vi "Unloading Sequence.vi"(8 "Abort":bool, 11 "Unload Button":bool) -> (0 "Not Start":bool)   [LabVIEW 2014]
uses:
  Unload State.ctl
  2015/2015 Master Code RECYCLE RUSH/Robot Global Data.vi
  Desired Arm Position.vi
panel:
  in  "Parameter":T1
  out "Turn 180":bool
  out "Close Arms":bool
  out "Open Arms":bool
  out "Lower Back Arms":bool
  out "Move Back":bool
  out "Raise Arms":bool
  out "Unload Front Arms":bool
  out "Start":bool
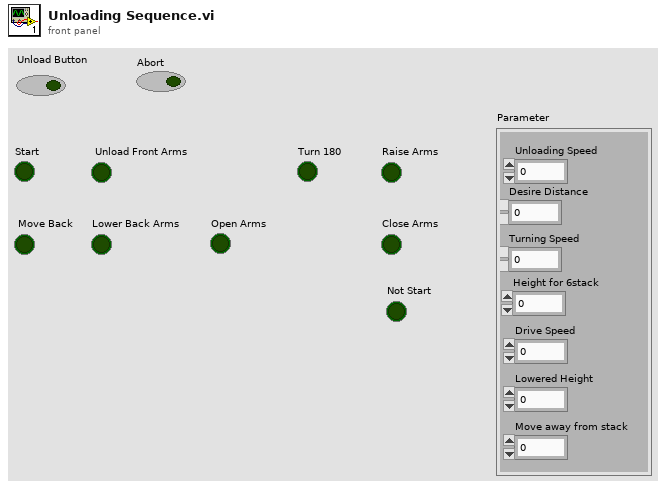
[diagram p1: front panel]
types:
  T1 = cluster{"Desire Distance  ":dbl, "Turning Speed":dbl, "Height for 6stack":dbl, "Drive Speed":dbl, "Lowered Height":dbl, "Move away from stack":dbl, "Unloading Speed":dbl}
  T2 = typedef "Unload State.ctl" = enum16{"Start", "Unload", "Back up", "Turn 180", "Raise Arms", "Move Back to S.P.", "Lower Back Arms", "Open Arms", "Back Up Before Drive", "Close Arms"}
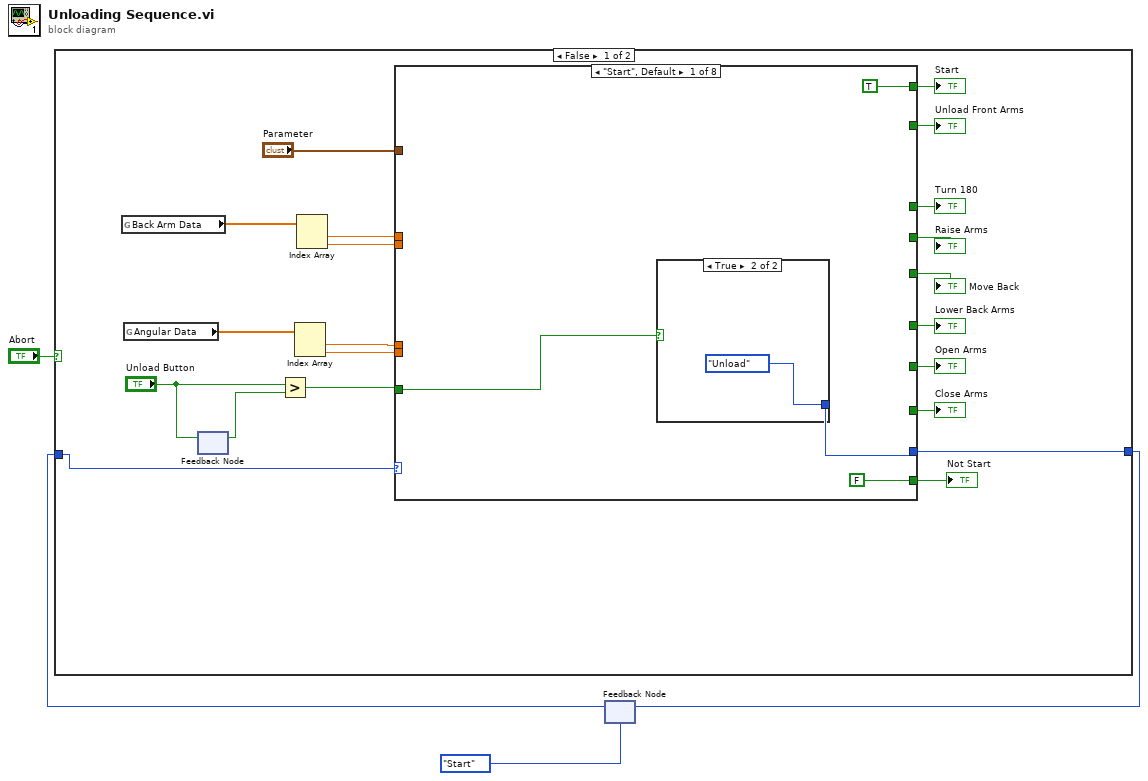
[diagram p0: block diagram]
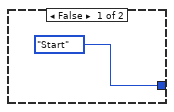
[diagram p2: hidden frame]
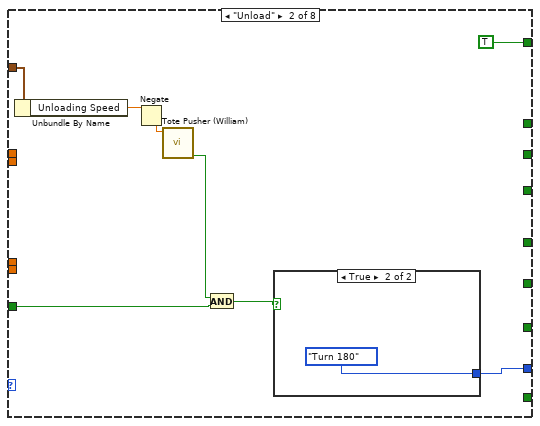
[diagram p3: hidden frame]
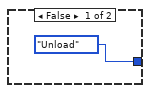
[diagram p4: hidden frame]
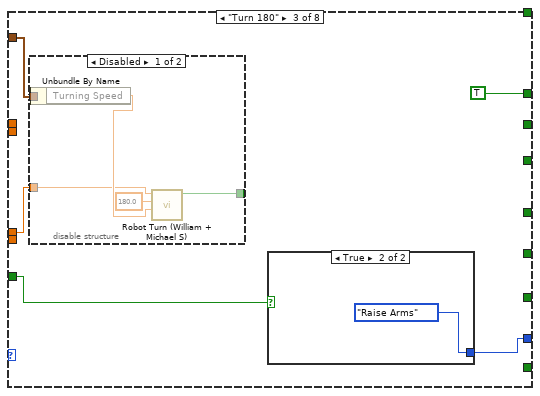
[diagram p5: hidden frame]
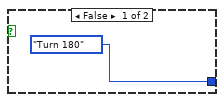
[diagram p7: hidden frame]
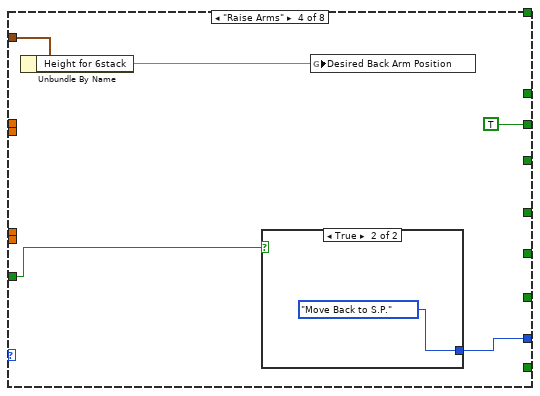
[diagram p8: hidden frame]
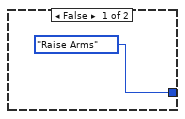
[diagram p9: hidden frame]
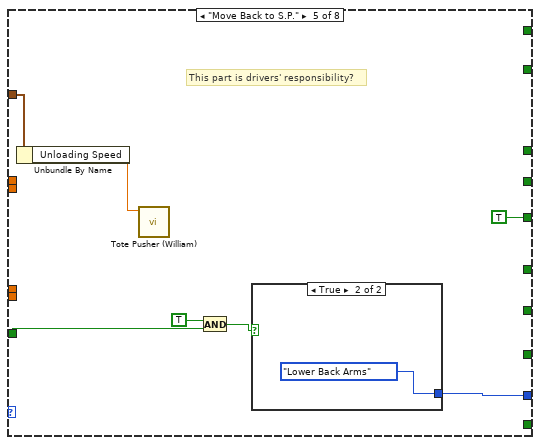
[diagram p10: hidden frame]
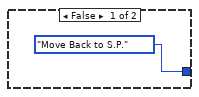
[diagram p11: hidden frame]
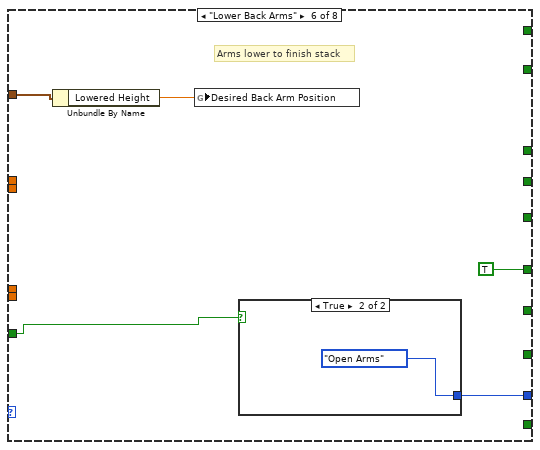
[diagram p12: hidden frame]
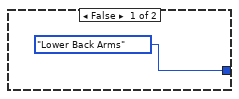
[diagram p13: hidden frame]
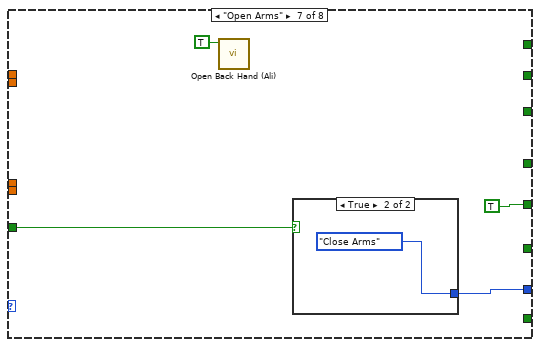
[diagram p14: hidden frame]
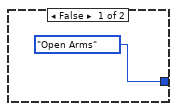
[diagram p15: hidden frame]
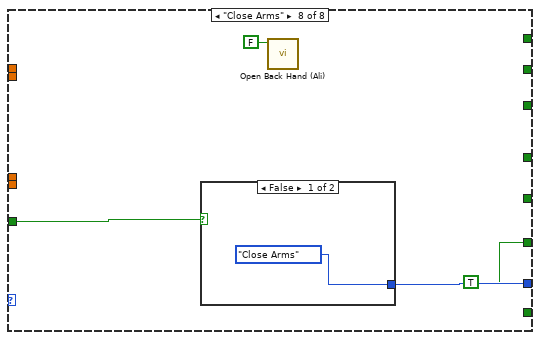
[diagram p16: hidden frame]
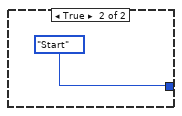
[diagram p17: hidden frame]
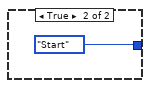
[diagram p18: hidden frame]
diagram:
  n1 = feedback #1(Unload_State."Start") -> (w2:T2)
  n2 = case shown="False" "Abort" {
    tunnel: [w7 Unload_State."Start"] -> w3
    tunnel: w2 -> [w6 _]
    frame False {
      n3 = global read "Robot Global Data.vi" "Back Arm Data"() -> (w13:dbl[])
      n4 = global read "Robot Global Data.vi" "Angular Data"() -> (w10:dbl[])
      n5 = feedback #2() -> (w18:bool)  [unwired: 1 in]
      n6 = feedback-in #2("Unload Button") -> ()
      n7 = Greater?(x="Unload Button", y=w18) -> (0:w17:bool)
      n8 = Index Array(array=w10) -> (element #1=w9:dbl, element #2=w8:dbl)  [unwired: 2 in]
      n9 = Index Array(array=w13) -> (element #1=w12:dbl, element #2=w11:dbl)  [unwired: 2 in]
      n10 = case shown="\"Start\", Default" w6 {
        tunnel: [TRUE _ _ _ _ _ _ _] -> w25
        tunnel: [_ TRUE _ _ _ _ _ _] -> w24
        tunnel: [_ _ _ _ _ _ _ TRUE] -> w23
        tunnel: [_ _ _ TRUE _ _ _ _] -> w22
        tunnel: [_ _ _ _ _ TRUE _ _] -> w21
        tunnel: [_ _ _ _ _ _ TRUE _] -> w20
        tunnel: w17 -> [w27 w37 w42 w54 w65 w70 w79 w86]
        tunnel: [w28 w38 w46 w58 w67 w74 w80 w85] -> w7
        tunnel: [_ _ TRUE _ _ _ _ _] -> w16
        tunnel: [_ _ _ _ TRUE _ _ _] -> w15
        tunnel: "Parameter" -> [_ w34 w44 w56 w63 w72 _ _]
        tunnel: w12 -> [_ _ _ _ _ _ _ _]
        tunnel: w11 -> [_ _ _ _ _ _ _ _]
        tunnel: w9 -> [_ _ w43 _ _ _ _ _]
        tunnel: w8 -> [_ _ _ _ _ _ _ _]
        tunnel: [FALSE _ _ _ _ _ _ _] -> w5
        frame "Start", Default {
          n11 = case shown="True" w27 {
            tunnel: [Unload_State."Start" Unload_State."Unload"] -> w28
            frame False {
            }
            frame True {
            }
          }
        }
        frame "Unload" {
          n12 = Unbundle By Name(w34) -> ("Unloading Speed"=w33:dbl)
          n13 = Negate(x=w33) -> (-x=w32:dbl)
          n14 = call "Tote Pusher (William).vi"("Motor Output"=w32) -> ("Pusher Out"=w36:bool)  [unwired: 9 in, 1 out]
          n15 = And(x=w36, y=w37) -> (x .and. y?=w35:bool)
          n16 = case shown="True" w35 {
            tunnel: [Unload_State."Unload" Unload_State."Turn 180"] -> w38
            frame False {
            }
            frame True {
            }
          }
        }
        frame "Turn 180" {
          n17 = disable-structure shown="Disabled" {
            disable-tunnel: [w50 _] -> _
            disable-tunnel: w44 -> [w49 _]
            disable-tunnel: w43 -> [w47 _]
            frame Disabled {
              n18 = Unbundle By Name(w49) -> ("Turning Speed"=w48:dbl)
              n19 = call "Robot Turn (William + Michael S).vi"("X axis value"=w48, "Desired Degree"=180.0, "Gyro Degrees"=w47) -> ("Stop"=w50:bool)  [unwired: 8 in]
            }
            frame Enabled {
            }
          }
          n20 = case shown="True" w42 {
            tunnel: [Unload_State."Turn 180" Unload_State."Raise Arms"] -> w46
            frame False {
            }
            frame True {
            }
          }
        }
        frame "Raise Arms" {
          n21 = Unbundle By Name(w56) -> ("Height for 6stack"=w55:dbl)
          n22 = case shown="True" w54 {
            tunnel: [Unload_State."Raise Arms" Unload_State."Move Back to S.P."] -> w58
            frame False {
            }
            frame True {
            }
          }
          n23 = global write "Desired Arm Position.vi" "Desired Back Arm Position"(w55) -> ()
        }
        frame "Move Back to S.P." {
          # "This part is drivers' responsibility?"
          n24 = Unbundle By Name(w63) -> ("Unloading Speed"=w62:dbl)
          n25 = call "Tote Pusher (William).vi"("Motor Output"=w62) -> ()  [unwired: 9 in, 2 out]
          n26 = And(x=TRUE, y=w65) -> (x .and. y?=w64:bool)
          n27 = case shown="True" w64 {
            tunnel: [Unload_State."Move Back to S.P." Unload_State."Lower Back Arms"] -> w67
            frame False {
            }
            frame True {
            }
          }
        }
        frame "Lower Back Arms" {
          # "Arms lower to finish stack"
          n28 = Unbundle By Name(w72) -> ("Lowered Height"=w71:dbl)
          n29 = global write "Desired Arm Position.vi" "Desired Back Arm Position"(w71) -> ()
          n30 = case shown="True" w70 {
            tunnel: [Unload_State."Lower Back Arms" Unload_State."Open Arms"] -> w74
            frame False {
            }
            frame True {
            }
          }
        }
        frame "Open Arms" {
          n31 = call "Open Back Hand (Ali).vi"("Open?"=TRUE) -> ()  [unwired: 11 in]
          n32 = case shown="True" w79 {
            tunnel: [Unload_State."Open Arms" Unload_State."Close Arms"] -> w80
            frame False {
            }
            frame True {
            }
          }
        }
        frame "Close Arms" {
          n33 = case shown="False" w86 {
            tunnel: [Unload_State."Close Arms" Unload_State."Start"] -> w85
            frame False {
            }
            frame True {
            }
          }
          n34 = call "Open Back Hand (Ali).vi"("Open?"=FALSE) -> ()  [unwired: 11 in]
        }
      }
      "Start" <- w25
      "Unload Front Arms" <- w24
      "Raise Arms" <- w22
      "Move Back" <- w15
      "Lower Back Arms" <- w21
      "Open Arms" <- w20
      "Close Arms" <- w23
      "Turn 180" <- w16
      "Not Start" <- w5
    }
    frame True {
    }
  }
  n35 = feedback-in #1(w3) -> ()
